vi "labelAlignment.vi"(8 "Error In":errorcluster, 11 "QwtScaleDraw In":refnum<class "QwtScaleDraw.lvclass">) -> (0 "Error Out":errorcluster, 2 "Value":T1=1 items=["AlignLeft"=1, "AlignRight"=2, "AlignHCenter"=4, "AlignJustify"=8, "AlignAbsolute"=16, "AlignHorizontal_Mask"=31, "AlignTop"=32, "AlignBottom"=64, "AlignVCenter"=128, "AlignBaseline"=256, "AlignVertical_Mask"=480, "AlignCenter"=132], 3 "QwtScaleDraw Out":refnum<class "QwtScaleDraw.lvclass">)   [LabVIEW 2014, in "QwtScaleDraw.lvclass"]
doc: "LabVIEW-specific documentation is not yet available. See <b>https://qwt.sourceforge.io/class_qwt_scale_draw.html#labelAlignment</b>"
uses:
  QwtScaleDraw.lvclass
  LQ Core/Qt/AlignmentFlag.ctl
  LQ Core/LQIdentity/LQIdentity.lvclass/LQIdentity.ctl
  LQ Core/LQ Core.lvlib
  LQ Core/LQIdentity/LQIdentity.lvclass
  LQ Core/Qt/Qt.lvlib
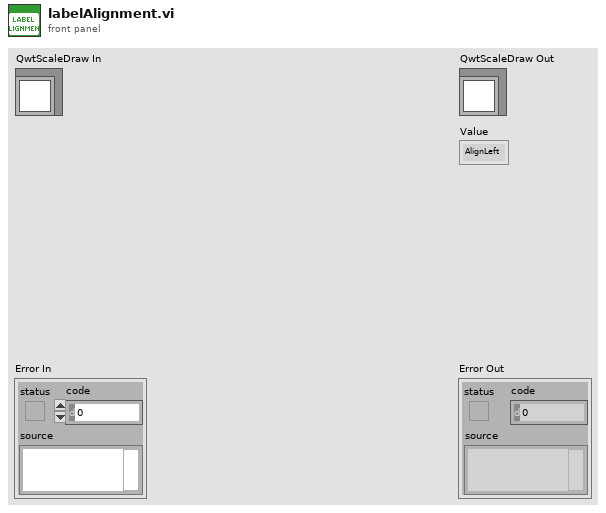
[diagram p1: front panel]
types:
  T1 = typedef "Qt.lvlib/AlignmentFlag.ctl" = i32
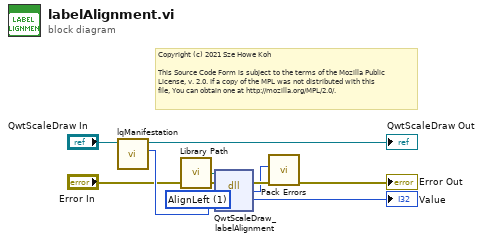
[diagram p0: block diagram]
diagram:
  w7 = T1 1 items=["AlignLeft"=1, "AlignRight"=2, "AlignHCenter"=4, "AlignJustify"=8, "AlignAbsolute"=16, "AlignHorizontal_Mask"=31, "AlignTop"=32, "AlignBottom"=64, "AlignVCenter"=128, "AlignBaseline"=256, "AlignVertical_Mask"=480, "AlignCenter"=132] ("retVal")
  # "Copyright (c) 2021 Sze Howe Koh\n\nThis Source Code Form is subject to the terms of the Mozilla Public\nLicense, v. 2.0. If a copy of the MPL was not distributed with this\nfile, You can obtain one at http://mozilla.org/MPL/2.0/."
  n1 = call "lqManifestation.vi"("LQIdentity in"="QwtScaleDraw In") -> ("Manifestation"=w5:u64, "LQIdentity out"=→"QwtScaleDraw Out":refnum<class "QwtScaleDraw.lvclass">)  [unwired: 9 in]
  n2 = call "Library Path.vi"() -> ("Library Path"=w6:path)
  n3 = dll-call lib="?" fn="QwtScaleDraw_labelAlignment"(path in=w6, error in="Error In", "_retVal"=w7, "_instance"=w5) -> (error out=w3:errorcluster, w1:i32, "_retVal"=→"Value":i32)  [unwired: 2 in, 1 out]
  n4 = call "Pack Errors.vi"("Error In"=w3, "Error Code"=w1) -> ("Error Out"=→"Error Out":errorcluster)  [unwired: 9 in]
